vi "Dis-en-able controls.vi"(8 "error in (no error)":errorcluster, 10 "State":T1(ring), 11 "Array":refnum<vi>[](array[refnum])) -> (0 "error out":errorcluster)   [LabVIEW 2015]
doc: "Enables, disables FP controls."
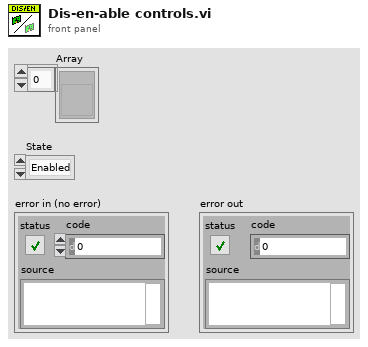
[diagram p1: front panel]
types:
  T1 = enum8{"Enabled", "Disabled", "Disabled and Grayed Out"}
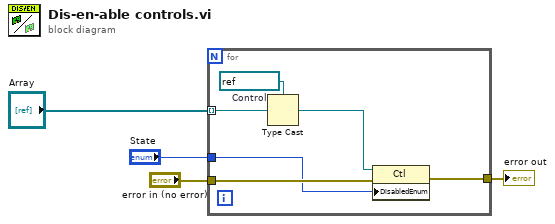
[diagram p0: block diagram]
diagram:
  n1 = for {
    tunnel: "Array" -> [w9] mode=indexing
    tunnel: [w7] -> w2
    tunnel: "error in (no error)" -> [w6]
    tunnel: "State" -> [w5]
    w10 = refnum<vi> refnum  # Control
    n2 = Type Cast(type=w10, x=w9) -> (*(type *) &x=w8:refnum<vi>)
    n3 = property class="Ctl"(reference=w8, error in=w6, "DisabledEnum"=w5) -> (error out=w7:errorcluster)  [unwired: 1 out]
  }
  "error out" <- w2
